vi "Read Height.vi"(8 "error in (no error)":errorcluster, 11 "Rect Collider in":refnum<class "Rect Collider.lvclass">) -> (0 "error out":errorcluster, 2 "Height":i16, 3 "Rect Collider out":refnum<class "Rect Collider.lvclass">)   [LabVIEW 2022 SP3, in "Rect Collider.lvclass"]
uses:
  Rect Collider.lvclass
  Rect Collider.lvclass/Rect Collider.ctl
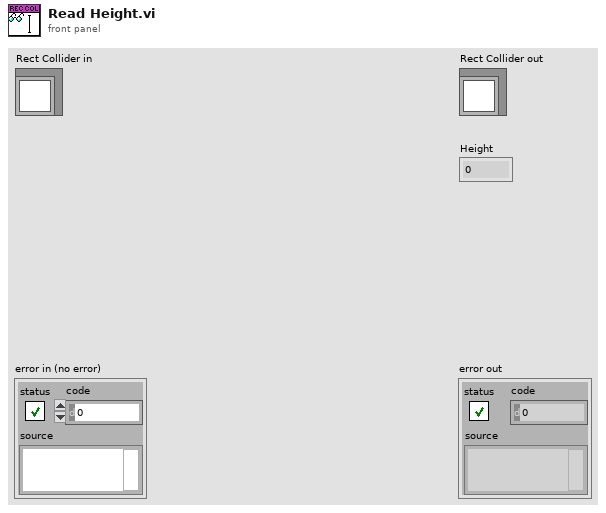
[diagram p1: front panel]
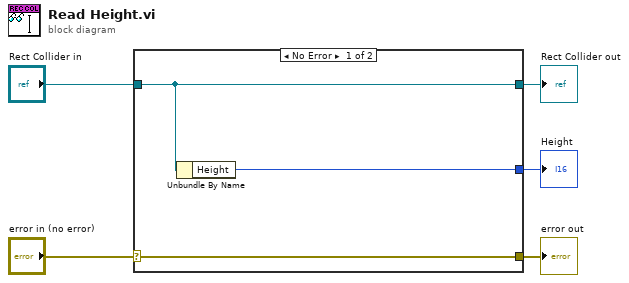
[diagram p0: block diagram]
diagram:
  n1 = case shown="No Error" "error in (no error)" {
    selector: "error in (no error)" -> [w8 w9]
    tunnel: [w8 w9] -> w4
    tunnel: [w7 w10] -> w2
    tunnel: "Rect Collider in" -> [w7 w10]
    tunnel: [w6 _] -> w1
    frame No Error {
      n2 = Unbundle By Name(w7) -> ("Height"=w6:i16)
    }
    frame Error {
    }
  }
  "error out" <- w4
  "Rect Collider out" <- w2
  "Height" <- w1
